vi "Find Serial Numbers.vi"() -> (3 "Array":T1[](array[typedef]))   [LabVIEW 2015]
uses:
  Resource Data.ctl
  <instrlib>/BK Precision 178XB Series/BK Precision 178XB Series.lvlib
panel:
  in  "Cluster 2":T1
  out "ID Query read buffer":string
  in  "Serial Configuration 2":T2={"Baud Rate (19200)"=19200, "Flow Control (1: XON/XOFF)"=1, "Termination Char (0:CR)"=0} {"Termination Char (0:CR)" items=["CR", "LF"]; "Flow Control (1: XON/XOFF)" items=["None", "XON/XOFF", "RTS/CTS (2701 Only)", "XON/XOFF & RTS/CTS (2701 Only)"]; "Baud Rate (19200)" items=["300"=300, "600"=600, "1200"=1200, "2400"=2400, "4800"=4800, "9600"=9600, "19.2k"=19200, "38.4k (2701 Only)"=38400, "57.6k (2701 Only)"=57600, "115.2k (2701 Only)"=115200]}
  in  "Serial Configuration":T3={"Baud Rate"=9600, "Parity"=0, "Data Bits"=8, "Stop Bits"=10} {"Stop Bits" items=["1.0"=10]; "Data Bits" items=["8"=8]; "Parity" items=["None", "Odd", "Even"]; "Baud Rate" items=["4800"=4800, "9600"=9600, "19200"=19200, "38400"=38400]}
  in  "Cluster":T1={"Resource"="ASRL3::INSTR", "Serial Number"="6474001036", "Model"=""}
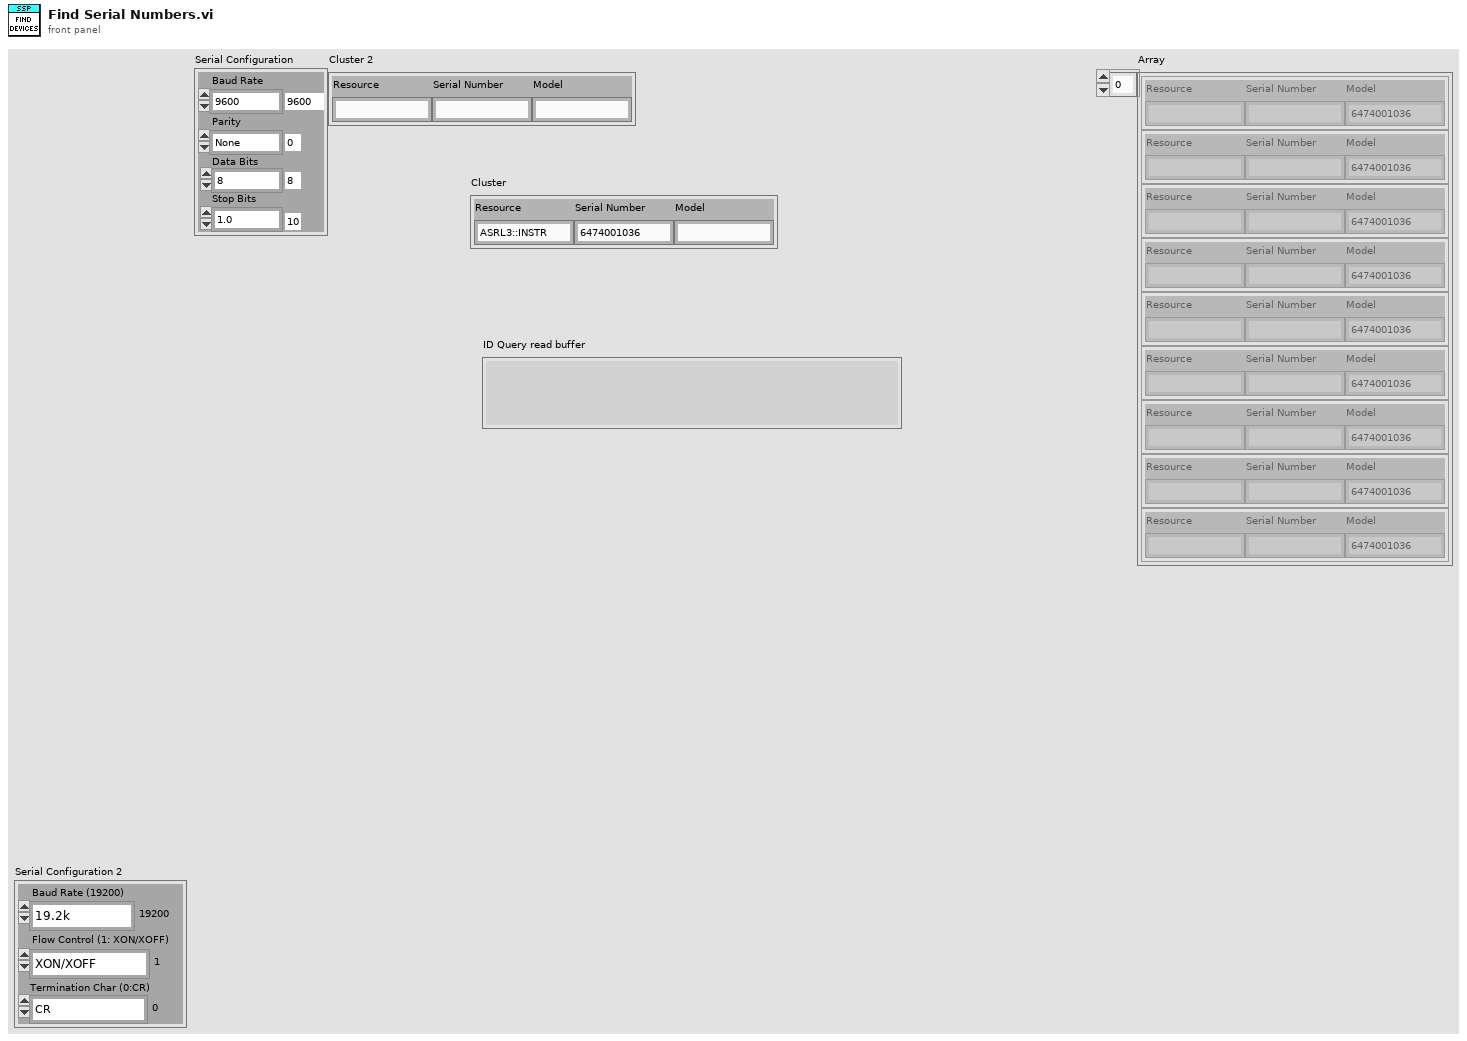
[diagram p1: front panel]
types:
  T1 = typedef "Resource Data.ctl" = cluster{"Resource":string, "Serial Number":string, "Model":string}
  T2 = cluster{"Baud Rate (19200)":u32, "Flow Control (1: XON/XOFF)":u16, "Termination Char (0:CR)":u16}
  T3 = cluster{"Baud Rate":u32, "Parity":u16, "Data Bits":u16, "Stop Bits":u16}
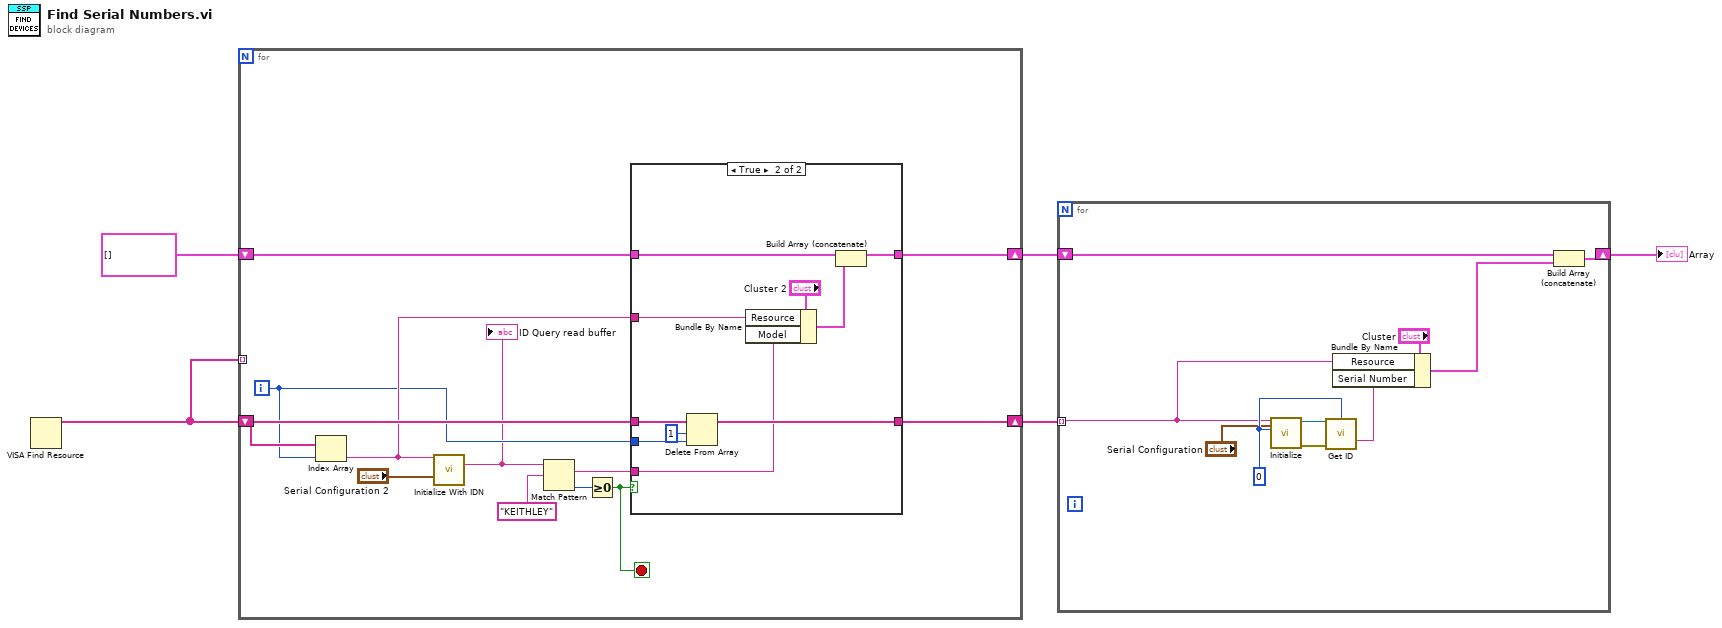
[diagram p0: block diagram]
diagram:
  n1 = VISA Find Resource() -> (3:w3:string[])  [unwired: 3 in, 2 out]
  n2 = for {
    shift-right: [w15] -> w5
    shift-left: w3 -> [w16]
    shift-right: [w12] -> w2
    shift-left: T1[] [] -> [w13]
    tunnel: w3 -> [_] mode=indexing
    i -> [w8]
    stop <- w10 stop-if-true
    n3 = Index Array(array=w16, index=w8) -> (element=w11:string)
    n4 = call "Initialize With IDN.vi"("VISA resource name"=w11, "Serial Configuration"="Serial Configuration 2") -> ("ID Query read buffer"=w7:string)  [unwired: 11 in, 2 out]
    "ID Query read buffer" <- w7
    n5 = Match Pattern(string=w7, regular expression="KEITHLEY") -> (match substring=w6:string, offset past match=w14:i32)  [unwired: 1 in, 2 out]
    n6 = Greater Or Equal To 0?(x=w14) -> (x >= 0?=w10:bool)
    n7 = case shown="True" w10 {
      tunnel: w16 -> [w19 w29]
      tunnel: [w19 w28] -> w15
      tunnel: w8 -> [_ w27]
      tunnel: w13 -> [w18 w25]
      tunnel: [w18 w24] -> w12
      tunnel: w6 -> [_ w21]
      tunnel: w11 -> [_ w20]
      frame False {
      }
      frame True {
        n8 = Delete From Array(array=w29, length=1, index=w27) -> (array with subset deleted=w28:string[])  [unwired: 1 out]
        n9 = Bundle By Name(cluster="Cluster 2", "Resource"=w20, "Model"=w21) -> (w23:T1)
        n10 = Build Array (concatenate)(w25, w23) -> (w24:T1[])
      }
    }
  }
  n11 = for {
    tunnel: w5 -> [w36] mode=indexing
    shift-right: [w31] -> w1
    shift-left: w2 -> [w32]
    w39 = u8 0 ("Communication Address (0)")
    n12 = call <instrlib>:"Initialize.vi"("Serial Configuration"="Serial Configuration", "Communication Address (0)"=w39, "VISA resource name"=w36) -> ("error out"=w33:errorcluster, "VISA resource name out"=w38:refnum<visa-resource-name>)  [unwired: 7 in]
    n13 = call <instrlib>:"Get ID.vi"("VISA resource name"=w38, "Communication Address (0)"=w39, "error in (no error)"=w33) -> ("Serial Number"=w35:string)  [unwired: 8 in, 4 out]
    n14 = Bundle By Name(cluster="Cluster", "Resource"=w36, "Serial Number"=w35) -> (w30:T1)
    n15 = Build Array (concatenate)(w32, w30) -> (w31:T1[])
  }
  "Array" <- w1
